vi "SetAxisParameter.vi"(8 "error in (no error)":errorcluster, 11 "DMC_1000B in":refnum<class "DMC_1000B.lvclass">) -> (0 "error out":errorcluster, 3 "DMC_1000B out":refnum<class "DMC_1000B.lvclass">)   [LabVIEW 2019, in "DMC_1000B.lvclass"]
uses:
  DMC_1000B.lvclass
  LLB/DMC1000B/Dmc1000/Dmc1000.lvlib
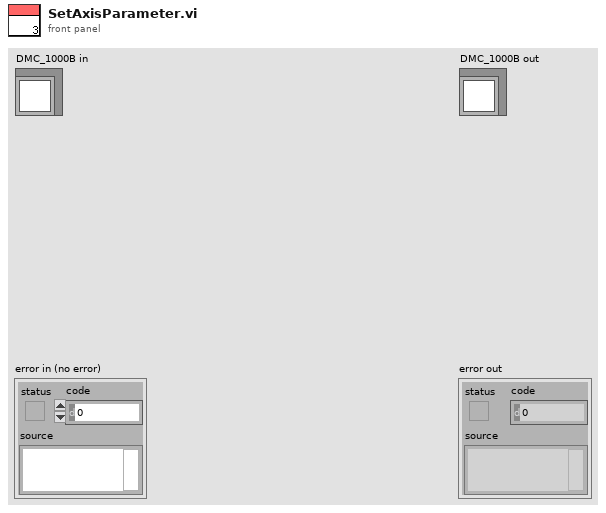
[diagram p1: front panel]
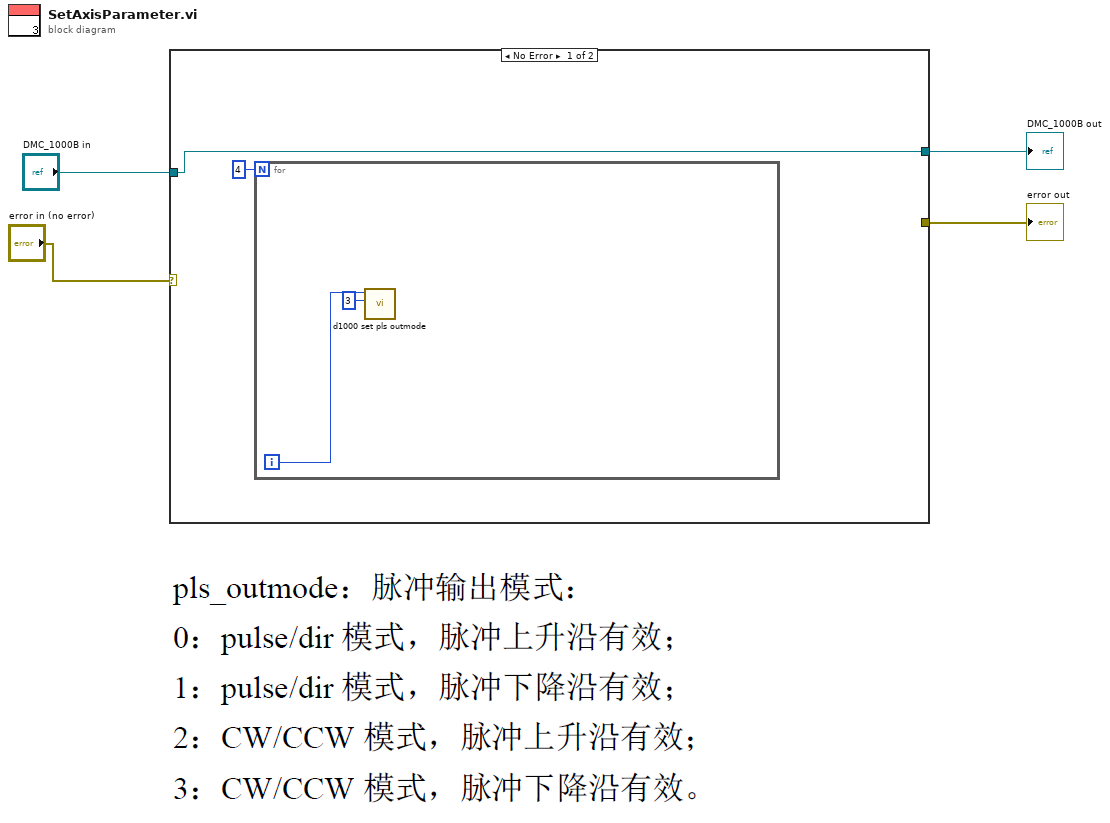
[diagram p0: block diagram]
diagram:
  n1 = case shown="No Error" "error in (no error)" {
    selector: "error in (no error)" -> [_ w9]
    tunnel: "DMC_1000B in" -> [w5 w10]
    tunnel: [w5 w10] -> w2
    tunnel: [_ w9] -> w1
    frame No Error {
      n2 = for {
        N: 4 -> [_]
        i -> [w8]
        n3 = call "d1000 set pls outmode.vi"("pls_outmode"=i16 3, "axis"=w8) -> ()  [unwired: 9 in, 1 out]
      }
    }
    frame Error {
    }
  }
  "error out" <- w1
  "DMC_1000B out" <- w2
